vi "Simplified example for blog.vi"() -> ()   [LabVIEW 2014]
panel:
  out "Quantity":i32[](array[numeric])=[1, 2, 3]
  out "Value":string[](array[string])=["£2", "£5", "£10"]
  out "Solutions":i32[][](array[numeric])
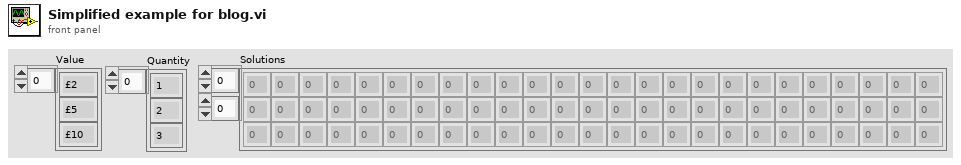
[diagram p1: front panel]
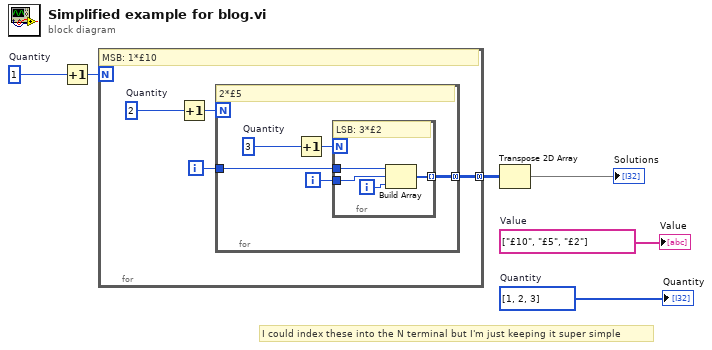
[diagram p0: block diagram]
diagram:
  w1 = i32[] [1, 2, 3]  # Quantity
  w2 = string[] ["£10", "£5", "£2"]  # Value
  w6 = 1  # Quantity
  # "I could index these into the N terminal but I'm just keeping it super simple"
  n1 = Increment(x=w6) -> (x+1=w5:i32)
  n2 = for {
    N: w5 -> [_]
    tunnel: [w9] -> w3 mode=concatenating
    i -> [w10]
    w7 = 2  # Quantity
    # "MSB: 1*£10"
    n3 = Increment(x=w7) -> (x+1=w8:i32)
    n4 = for {
      N: w8 -> [_]
      tunnel: w10 -> [w14]
      tunnel: [w13] -> w9 mode=concatenating
      i -> [w15]
      w11 = 3  # Quantity
      # "2*£5"
      n5 = Increment(x=w11) -> (x+1=w12:i32)
      n6 = for {
        N: w12 -> [_]
        tunnel: w15 -> [w18]
        tunnel: w14 -> [w17]
        tunnel: [w16] -> w13 mode=indexing
        i -> [w19]
        # "LSB: 3*£2"
        n7 = Build Array(w17, w18, w19) -> (w16:i32[])
      }
    }
  }
  n8 = Transpose 2D Array(2D array=w3) -> (transposed array=→"Solutions":i32[][])
  "Value" <- w2
  "Quantity" <- w1
